vi "UdCounter_RegisterLVEvent.vi"(3 "UdCntrEvent":refnum<user-event>, 4 "error in (no error)":errorcluster, 5 "Task ID":u32) -> (0 "UdCntrEvent":refnum<user-event>, 1 "error out":errorcluster, 2 "Task ID out":u32)   [LabVIEW 2015]
uses:
  Windows/System32/AdvLvDaq.dll
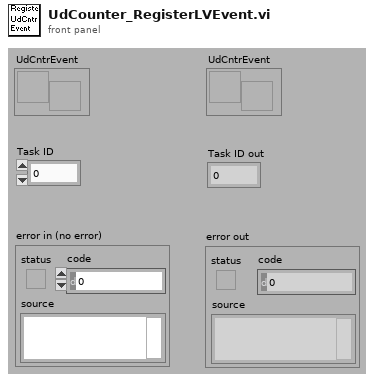
[diagram p1: front panel]
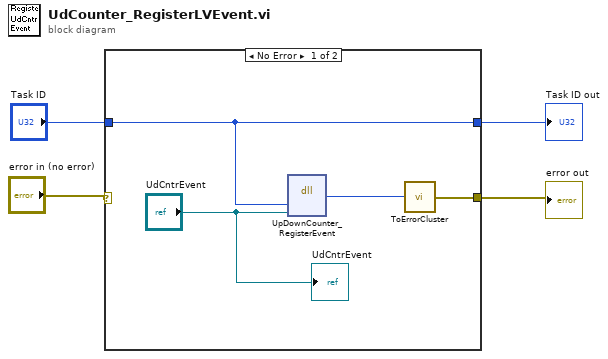
[diagram p0: block diagram]
diagram:
  n1 = case shown="No Error" "error in (no error)" {
    selector: "error in (no error)" -> [_ w10]
    tunnel: [w7 w10] -> w3
    tunnel: "Task ID" -> [w6 w9]
    tunnel: [w6 w9] -> w1
    frame No Error {
      n2 = dll-call lib="C:/Windows/System32/AdvLvDaq.dll" fn="UpDownCounter_RegisterEvent"("taskID"=w6, "eventRef"="UdCntrEvent") -> ("return type"=w8:i32)  [unwired: 4 in, 3 out]
      n3 = call "ToErrorCluster.vi"("error code"=w8) -> ("error out"=w7:errorcluster)
      "UdCntrEvent" <- "UdCntrEvent"
    }
    frame Error {
    }
  }
  "error out" <- w3
  "Task ID out" <- w1
